vi "Simulated WF.vi"(8 "error in (no error)":errorcluster) -> (0 "error out":errorcluster, 3 "signal out":waveform(dbl))   [LabVIEW 2020]
uses:
  <vilib>/measure/NI_MABase.lvlib
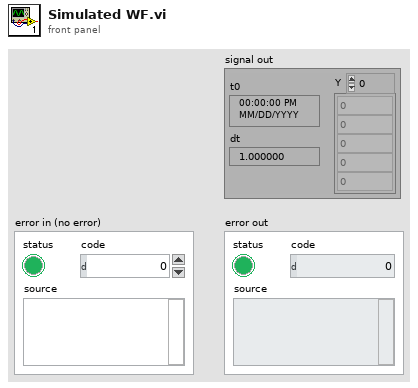
[diagram p1: front panel]
types:
  T1 = enum16{"Sine Wave", "Triangle Wave", "Square Wave", "Sawtooth Wave"}
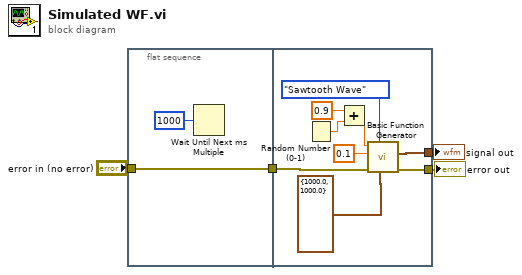
[diagram p0: block diagram]
diagram:
  n1 = flat-sequence {
    tunnel: "error in (no error)" -> [w6]
    tunnel: [w6] -> w4
    tunnel: [w15] -> w3
    tunnel: [w12] -> w2
    tunnel: w4 -> [w11]
    frame #0 {
      n2 = Wait Until Next ms Multiple(millisecond multiple=u32 1000) -> ()  [unwired: 1 out]
    }
    frame #1 {
      n3 = Random Number (0-1)() -> (number: 0 to 1=w14:dbl)
      n4 = Add(x=0.9 ("frequency"), y=w14) -> (x+y=w13:dbl)
      n5 = call <vilib>:"Basic Function Generator.vi"("sampling info"=cluster{"Fs":dbl, "#s":dbl} {"Fs"=1000.0, "#s"=1000.0}, "signal type"=T1."Sawtooth Wave", "error in (no error)"=w11, "amplitude"=0.1, "frequency"=w13) -> ("error out"=w12:errorcluster, "signal out"=w15:waveform(dbl))  [unwired: 4 in, 1 out]
    }
  }
  "signal out" <- w3
  "error out" <- w2
